vi "calculate starts.vi"(0 "Tomo in":refnum<class "Tomo.lvclass">, 11 "error in (no error)":errorcluster) -> (3 "x loop number":i32, 4 "Tomo out":refnum<class "Tomo.lvclass">, 6 "x_start":dbl[unit], 8 "y_start":dbl[unit], 10 "pretomo step size (px)":dbl, 14 "y loop number":i32, 15 "error out":errorcluster)   [LabVIEW 2012, in "Tomo.lvclass"]
uses:
  Tomo.lvclass
  Tomo.lvclass/Tomo.ctl
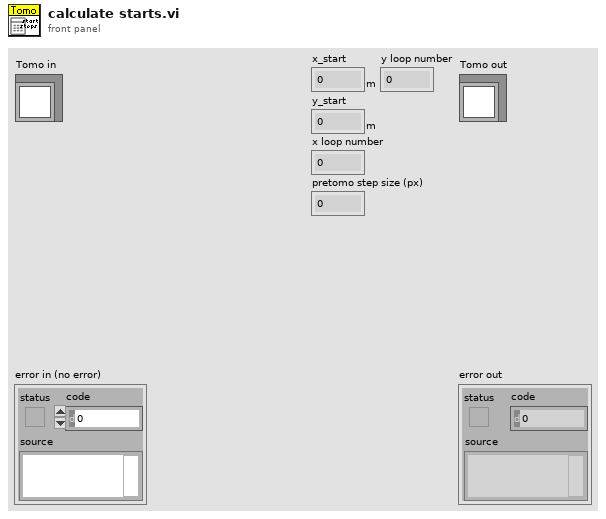
[diagram p1: front panel]
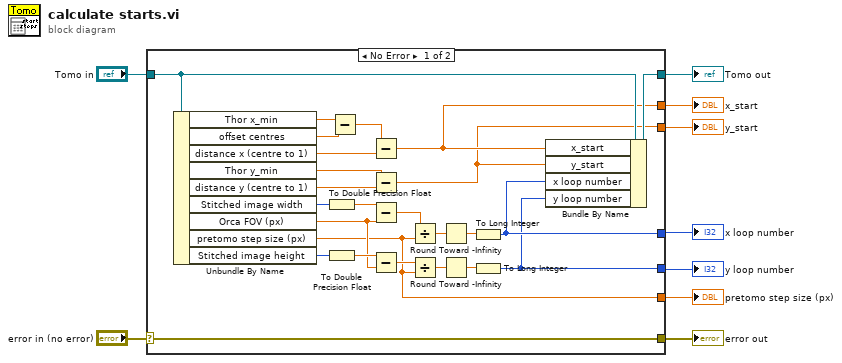
[diagram p0: block diagram]
diagram:
  n1 = case shown="No Error" "error in (no error)" {
    selector: "error in (no error)" -> [w34 w36]
    tunnel: [w34 w36] -> w8
    tunnel: [w28 w35] -> w6
    tunnel: "Tomo in" -> [w29 w35]
    tunnel: [w25 _] -> w5
    tunnel: [w23 _] -> w4
    tunnel: [w12 _] -> w3
    tunnel: [w11 _] -> w2
    tunnel: [w10 _] -> w1
    frame No Error {
      n2 = Unbundle By Name(w29) -> ("Thor x_min"=w32:dbl[unit], "offset centres"=w33:dbl[unit], "distance x (centre to 1)"=w30:dbl[unit], "Thor y_min"=w27:dbl[unit], "distance y (centre to 1)"=w26:dbl[unit], "Stitched image width"=w24:i32, "Orca FOV (px)"=w16:dbl, "pretomo step size (px)"=w10:dbl, "Stitched image height"=w18:i32)
      n3 = To Double Precision Float(number=w24) -> (double precision float=w22:dbl)
      n4 = To Double Precision Float(number=w18) -> (double precision float=w17:dbl)
      n5 = Subtract(x=w32, y=w33) -> (x-y=w31:dbl[unit])
      n6 = Subtract(x=w31, y=w30) -> (x-y=w25:dbl[unit])
      n7 = Subtract(x=w27, y=w26) -> (x-y=w23:dbl[unit])
      n8 = Subtract(x=w22, y=w16) -> (x-y=w21:dbl)
      n9 = Subtract(x=w17, y=w16) -> (x-y=w13:dbl)
      n10 = Divide(x=w21, y=w10) -> (x/y=w20:dbl)
      n11 = Divide(x=w13, y=w10) -> (x/y=w14:dbl)
      n12 = Round Toward -Infinity(1:w20) -> (0:w19:dbl)
      n13 = Round Toward -Infinity(1:w14) -> (0:w15:dbl)
      n14 = To Long Integer(number=w19) -> (32bit integer=w12:i32)
      n15 = To Long Integer(number=w15) -> (32bit integer=w11:i32)
      n16 = Bundle By Name(cluster=w29, "x_start"=w25, "y_start"=w23, "x loop number"=w12, "y loop number"=w11) -> (w28:refnum<class "Tomo.lvclass">)
    }
    frame Error {
    }
  }
  "error out" <- w8
  "Tomo out" <- w6
  "x_start" <- w5
  "y_start" <- w4
  "x loop number" <- w3
  "y loop number" <- w2
  "pretomo step size (px)" <- w1
